vi "Align Buffers.vi"(8 "error in (no error)":errorcluster, 10 "base Buffers":refnum<class "Buffers.lvclass">, 11 "Buffers in":refnum<class "Buffers.lvclass">) -> (0 "error out":errorcluster, 3 "Buffers out":refnum<class "Buffers.lvclass">)   [LabVIEW 2017, in "DSF Core.lvlib" / "Buffers.lvclass"]
uses:
  Buffers.lvclass
  Buffers.lvclass/Buffers.ctl
  Buffer.lvclass
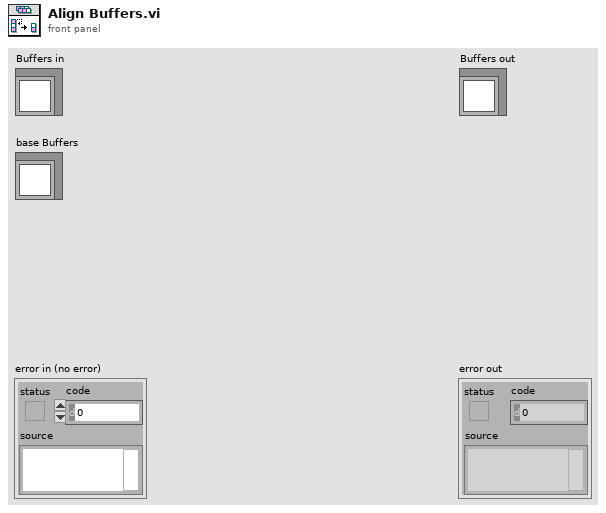
[diagram p1: front panel]
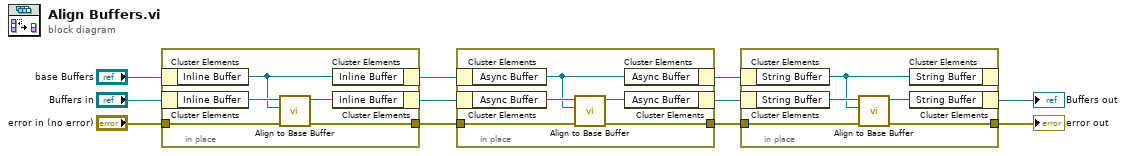
[diagram p0: block diagram]
diagram:
  n1 = in-place {
    in-place-border: "error in (no error)" -> [w14]
    in-place-border: [w13] -> w8
    n2 = in-place-cluster #1("base Buffers") -> ("Inline Buffer"=w12:refnum<class "Buffer.lvclass">)
    n3 = in-place-cluster #2("Buffers in") -> ("Inline Buffer"=w16:refnum<class "Buffer.lvclass">)
    n4 = call "Align to Base Buffer.vi"("error in (no error)"=w14, "base Buffer"=w12, "Buffer in"=w16) -> ("error out"=w13:errorcluster, "Buffer out"=w15:refnum<class "Buffer.lvclass">)  [unwired: 7 in]
    n5 = in-place-cluster #1("Inline Buffer"=w12) -> (w5:refnum<class "Buffers.lvclass">)
    n6 = in-place-cluster #2("Inline Buffer"=w15) -> (w6:refnum<class "Buffers.lvclass">)
  }
  n7 = in-place {
    in-place-border: w8 -> [w19]
    in-place-border: [w18] -> w7
    n8 = in-place-cluster #3(w5) -> ("Async Buffer"=w17:refnum<class "Buffer.lvclass">)
    n9 = in-place-cluster #4(w6) -> ("Async Buffer"=w21:refnum<class "Buffer.lvclass">)
    n10 = call "Align to Base Buffer.vi"("error in (no error)"=w19, "base Buffer"=w17, "Buffer in"=w21) -> ("error out"=w18:errorcluster, "Buffer out"=w20:refnum<class "Buffer.lvclass">)  [unwired: 7 in]
    n11 = in-place-cluster #3("Async Buffer"=w17) -> (w3:refnum<class "Buffers.lvclass">)
    n12 = in-place-cluster #4("Async Buffer"=w20) -> (w4:refnum<class "Buffers.lvclass">)
  }
  n13 = in-place {
    in-place-border: w7 -> [w24]
    in-place-border: [w23] -> w2
    n14 = in-place-cluster #5(w3) -> ("String Buffer"=w22:refnum<class "Buffer.lvclass">)
    n15 = in-place-cluster #6(w4) -> ("String Buffer"=w26:refnum<class "Buffer.lvclass">)
    n16 = call "Align to Base Buffer.vi"("error in (no error)"=w24, "base Buffer"=w22, "Buffer in"=w26) -> ("error out"=w23:errorcluster, "Buffer out"=w25:refnum<class "Buffer.lvclass">)  [unwired: 7 in]
    n17 = in-place-cluster #5("String Buffer"=w22) -> ()  [unwired: 1 out]
    n18 = in-place-cluster #6("String Buffer"=w25) -> (→"Buffers out":refnum<class "Buffers.lvclass">)
  }
  "error out" <- w2
